vi "Set cif_manager_PluginStatus.vi"(7 "Complete Call (T)":bool=TRUE, 8 "error in (no error)":errorcluster, 10 "package_templatemessage":T1, 11 "gRPCid":T16) -> (0 "error out":errorcluster)   [LabVIEW 2021, in "CIF_Manager_server.lvlib"]
uses:
  CIF_Manager_server.lvlib
  <vilib>/gRPC/LabVIEW gRPC Library/Shared/grpcId.ctl
  cif_manager_PluginStatus.ctl
  cif_manager_PluginName.ctl
  cif_plugincore_StatusData.ctl
  cif_plugincore_StatusData_PluginState.ctl
  cif_plugincore_TimingStatistics.ctl
  cif_common_TimingStats.ctl
  cif_plugincore_FifoStatistics.ctl
  cif_plugincore_Error.ctl
  cif_plugincore_MonitorDoubles.ctl
  cif_plugincore_MonitorU64.ctl
  cif_plugincore_MonitorI64.ctl
  cif_channelcore_Channels.ctl
  cif_channelcore_Channel.ctl
  cif_channelcore_ChannelDirection.ctl
  cif_channelcore_ChannelPattern.ctl
  cif_manager_PluginStatus_Flat.ctl
  cif_manager_PluginName_Flat.ctl
  cif_plugincore_StatusData_Flat.ctl
  cif_plugincore_TimingStatistics_Flat.ctl
  cif_common_TimingStats_Flat.ctl
  cif_plugincore_FifoStatistics_Flat.ctl
  cif_plugincore_Error_Flat.ctl
  cif_plugincore_MonitorDoubles_Flat.ctl
  cif_plugincore_MonitorU64_Flat.ctl
  cif_plugincore_MonitorI64_Flat.ctl
  cif_channelcore_Channels_Flat.ctl
  cif_channelcore_Channel_Flat.ctl
  dcc74a39-081a-4bdd-860b-8ed792803c96.vi
  <vilib>/gRPC/LabVIEW gRPC Library/Shared/TranslateGrpcError.vi
  RichToFlatcif_manager_PluginName.vi
  RichToFlatcif_plugincore_StatusData.vi
  RichToFlatcif_channelcore_Channels.vi
  RichToFlatcif_plugincore_TimingStatistics.vi
  RichToFlatcif_plugincore_FifoStatistics.vi
  RichToFlatcif_plugincore_Error.vi
  RichToFlatcif_plugincore_MonitorDoubles.vi
  RichToFlatcif_plugincore_MonitorU64.vi
  RichToFlatcif_plugincore_MonitorI64.vi
  RichToFlatcif_channelcore_Channel.vi
  RichToFlatcif_common_TimingStats.vi
  <vilib>/gRPC/LabVIEW gRPC Library/Server API/Server/Get Server DLL Path.vi
  <vilib>/Utility/error.llb/Error Cluster From Error Code.vi
  <vilib>/gRPC/LabVIEW gRPC Library/grpc-lvsupport-release.lvlib
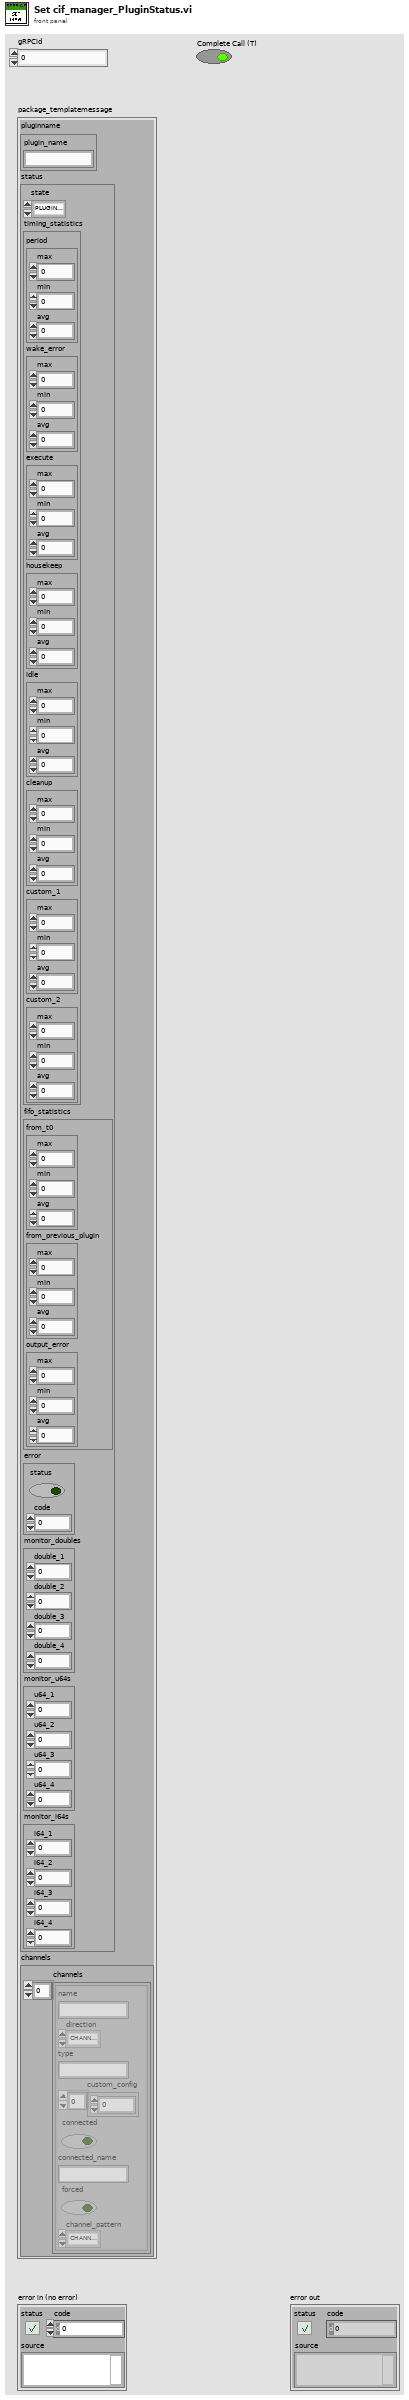
[diagram p1: front panel]
types:
  T1 = typedef "CIF_Manager_server.lvlib/cif_manager_PluginStatus.ctl" = cluster{"pluginname":T2, "status":T3, "channels":T12}
  T2 = typedef "CIF_Manager_server.lvlib/cif_manager_PluginName.ctl" = cluster{"plugin_name":string}
  T3 = typedef "CIF_Manager_server.lvlib/cif_plugincore_StatusData.ctl" = cluster{"state":T4, "timing_statistics":T5, "fifo_statistics":T7, "error":T8, "monitor_doubles":T9, "monitor_u64s":T10, "monitor_i64s":T11}
  T4 = typedef "CIF_Manager_server.lvlib/cif_plugincore_StatusData_PluginState.ctl" = enum32{"PLUGINSTATE_UNKNOWN", "PLUGINSTATE_CREATING", "PLUGINSTATE_LISTENING", "PLUGINSTATE_RUNNING", "PLUGINSTATE_CLEANINGUP", "PLUGINSTATE_DESTROYING"}
  T5 = typedef "CIF_Manager_server.lvlib/cif_plugincore_TimingStatistics.ctl" = cluster{"period":T6, "wake_error":T6, "execute":T6, "housekeep":T6, "idle":T6, "cleanup":T6, "custom_1":T6, "custom_2":T6}
  T6 = typedef "CIF_Manager_server.lvlib/cif_common_TimingStats.ctl" = cluster{"max":i64, "min":i64, "avg":dbl}
  T7 = typedef "CIF_Manager_server.lvlib/cif_plugincore_FifoStatistics.ctl" = cluster{"from_t0":T6, "from_previous_plugin":T6, "output_error":T6}
  T8 = typedef "CIF_Manager_server.lvlib/cif_plugincore_Error.ctl" = cluster{"status":bool, "code":i32}
  T9 = typedef "CIF_Manager_server.lvlib/cif_plugincore_MonitorDoubles.ctl" = cluster{"double_1":dbl, "double_2":dbl, "double_3":dbl, "double_4":dbl}
  T10 = typedef "CIF_Manager_server.lvlib/cif_plugincore_MonitorU64.ctl" = cluster{"u64_1":u64, "u64_2":u64, "u64_3":u64, "u64_4":u64}
  T11 = typedef "CIF_Manager_server.lvlib/cif_plugincore_MonitorI64.ctl" = cluster{"i64_1":i64, "i64_2":i64, "i64_3":i64, "i64_4":i64}
  T12 = typedef "CIF_Manager_server.lvlib/cif_channelcore_Channels.ctl" = cluster{"channels":T13[]}
  T13 = typedef "CIF_Manager_server.lvlib/cif_channelcore_Channel.ctl" = cluster{"name":string, "direction":T14, "type":string, "custom_config":u8[], "connected":bool, "connected_name":string, "forced":bool, "channel_pattern":T15}
  T14 = typedef "CIF_Manager_server.lvlib/cif_channelcore_ChannelDirection.ctl" = enum32{"CHANNELDIRECTION_UNKNOWN", "CHANNELDIRECTION_PUBLISHER", "CHANNELDIRECTION_SUBSCRIBER"}
  T15 = typedef "CIF_Manager_server.lvlib/cif_channelcore_ChannelPattern.ctl" = enum32{"CHANNELPATTERN_UNKNOWN", "CHANNELPATTERN_TAG", "CHANNELPATTERN_FIFO", "CHANNELPATTERN_MULTIFIFO", "CHANNELPATTERN_BACKPRESSUREFIFO"}
  T16 = typedef "grpc-lvsupport-release.lvlib/grpcId.ctl" = u64
  T17 = typedef "CIF_Manager_server.lvlib/cif_manager_PluginStatus_Flat.ctl" = cluster{"pluginname":T18, "status":T19, "channels":T27}
  T18 = typedef "CIF_Manager_server.lvlib/cif_manager_PluginName_Flat.ctl" = cluster{"plugin_name":string}
  T19 = typedef "CIF_Manager_server.lvlib/cif_plugincore_StatusData_Flat.ctl" = cluster{"state":T4, "timing_statistics":T20, "fifo_statistics":T22, "error":T23, "monitor_doubles":T24, "monitor_u64s":T25, "monitor_i64s":T26}
  T20 = typedef "CIF_Manager_server.lvlib/cif_plugincore_TimingStatistics_Flat.ctl" = cluster{"period":T21, "wake_error":T21, "execute":T21, "housekeep":T21, "idle":T21, "cleanup":T21, "custom_1":T21, "custom_2":T21}
  T21 = typedef "CIF_Manager_server.lvlib/cif_common_TimingStats_Flat.ctl" = cluster{"max":i64, "min":i64, "avg":dbl}
  T22 = typedef "CIF_Manager_server.lvlib/cif_plugincore_FifoStatistics_Flat.ctl" = cluster{"from_t0":T21, "from_previous_plugin":T21, "output_error":T21}
  T23 = typedef "CIF_Manager_server.lvlib/cif_plugincore_Error_Flat.ctl" = cluster{"status":bool, "code":i32}
  T24 = typedef "CIF_Manager_server.lvlib/cif_plugincore_MonitorDoubles_Flat.ctl" = cluster{"double_1":dbl, "double_2":dbl, "double_3":dbl, "double_4":dbl}
  T25 = typedef "CIF_Manager_server.lvlib/cif_plugincore_MonitorU64_Flat.ctl" = cluster{"u64_1":u64, "u64_2":u64, "u64_3":u64, "u64_4":u64}
  T26 = typedef "CIF_Manager_server.lvlib/cif_plugincore_MonitorI64_Flat.ctl" = cluster{"i64_1":i64, "i64_2":i64, "i64_3":i64, "i64_4":i64}
  T27 = typedef "CIF_Manager_server.lvlib/cif_channelcore_Channels_Flat.ctl" = cluster{"channels":T28[]}
  T28 = typedef "CIF_Manager_server.lvlib/cif_channelcore_Channel_Flat.ctl" = cluster{"name":string, "direction":T14, "type":string, "custom_config":u8[], "connected":bool, "connected_name":string, "forced":bool, "channel_pattern":T15}
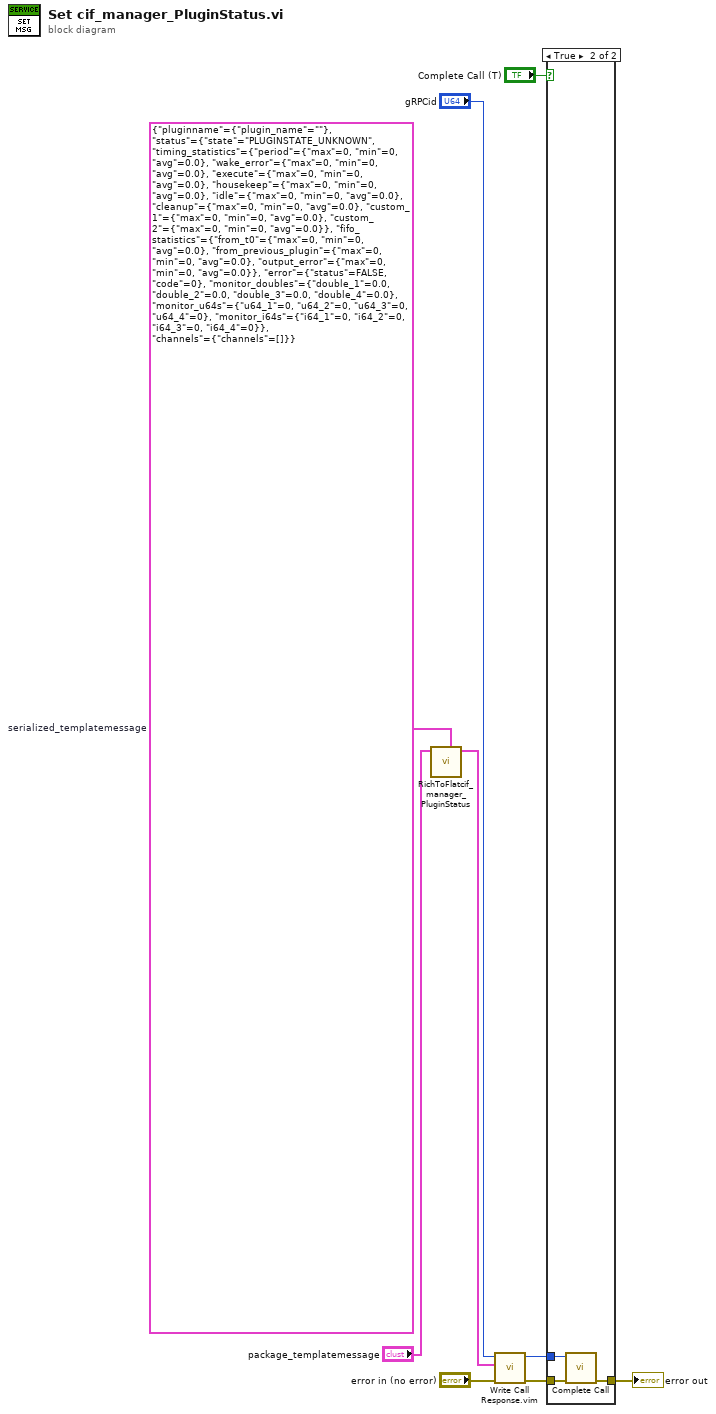
[diagram p0: block diagram]
diagram:
  w2 = T17 {"pluginname"={"plugin_name"=""}, "status"={"state"=enum."PLUGINSTATE_UNKNOWN", "timing_statistics"={"period"={"max"=0, "min"=0, "avg"=0.0}, "wake_error"={"max"=0, "min"=0, "avg"=0.0}, "execute"={"max"=0, "min"=0, "avg"=0.0}, "housekeep"={"max"=0, "min"=0, "avg"=0.0}, "idle"={"max"=0, "min"=0, "avg"=0.0}, "cleanup"={"max"=0, "min"=0, "avg"=0.0}, "custom_1"={"max"=0, "min"=0, "avg"=0.0}, "custom_2"={"max"=0, "min"=0, "avg"=0.0}}, "fifo_statistics"={"from_t0"={"max"=0, "min"=0, "avg"=0.0}, "from_previous_plugin"={"max"=0, "min"=0, "avg"=0.0}, "output_error"={"max"=0, "min"=0, "avg"=0.0}}, "error"={"status"=FALSE, "code"=0}, "monitor_doubles"={"double_1"=0.0, "double_2"=0.0, "double_3"=0.0, "double_4"=0.0}, "monitor_u64s"={"u64_1"=0, "u64_2"=0, "u64_3"=0, "u64_4"=0}, "monitor_i64s"={"i64_1"=0, "i64_2"=0, "i64_3"=0, "i64_4"=0}}, "channels"={"channels"=[]}}  # serialized_templatemessage
  n1 = call "RichToFlatcif_manager_PluginStatus.vi"("OutputClusterType"=w2, "InputCluster"="package_templatemessage") -> ("OutputCluster"=w1:T17)  [unwired: 9 in]
  n2 = call "Write Call Response.vim"("error in"="error in (no error)", "Response Data"=w1, "gRPCid in"="gRPCid") -> ("error out"=w6:errorcluster, "gRPCid out"=w7:T16)  [unwired: 7 in]
  n3 = case shown="True" "Complete Call (T)" {
    tunnel: [w10 w13] -> w9
    tunnel: w7 -> [_ w12]
    tunnel: w6 -> [w10 w11]
    frame False {
    }
    frame True {
      n4 = call <vilib>:"Complete Call.vi"("gRPCid"=w12, "error in"=w11) -> ("error out"=w13:errorcluster)  [unwired: 8 in]
    }
  }
  "error out" <- w9
